vi "TL_init_sCMOS_for_scan.vi"(7 "queue sCMOS":refnum<queue>, 8 "error in":errorcluster, 9 "data":cluster{"Channel":string, "ROI #":i32}, 10 "Channel #":i32, 11 "Time lapse parameters":T2) -> (0 "error out":errorcluster)   [LabVIEW 2015]
uses:
  CONTROLS/Q_camera_element.ctl
  CONTROLS/Q_main_element.ctl
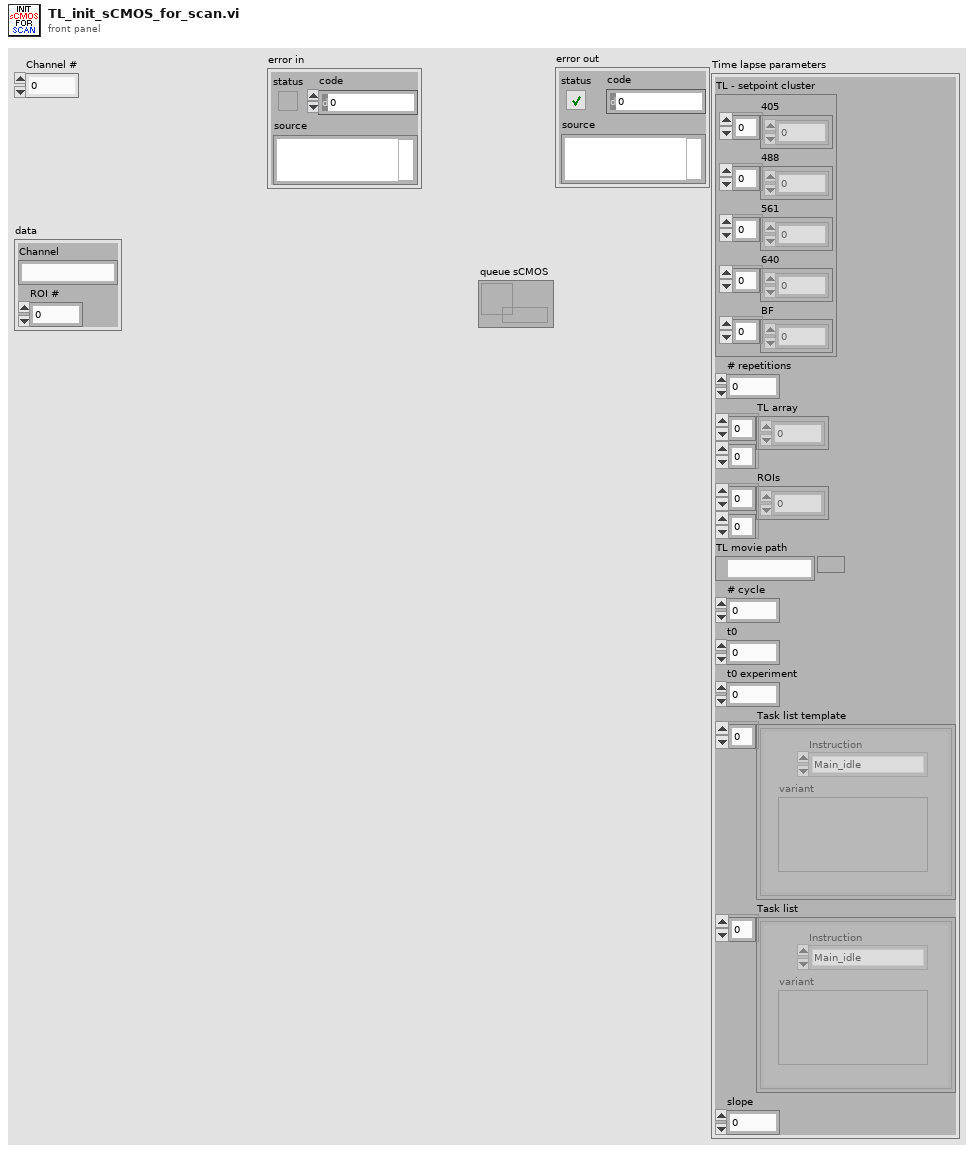
[diagram p1: front panel]
types:
  T1 = typedef "Q_main_element.ctl" = cluster{"variant":variant, "Instruction":enum16{"Main_idle", "Main_initialize", "Main_error", "Main_DAQ_initialization_results", "Main_ASI_initialization_results", "Main_Piezo_initialization_results", "Main_Valve_initialization_results", "Main_Pump_initialization_results", "Main_CAMERA_initialization_results", "Main_DAQ_error", "Main_ASI_error", "Main_Piezo_error", "Main_CAMERA_error", "Main_Valve_error", "Main_Pump_error", "Main_start_acquiring", "Main_not_acquiring", "Main_acquiring", "Main_stop_acquiring", "Main_change_exposure", "Main_define_ROI", "Main_read_kinetic_time", "Main_cooler", "Main_read_temperature", "Main_save_XY", "Main_load_XY", "Main_discard_XY", "Main_move_to_XY", "Main_measure_QPD", "Main_autofocus_calibration", "Main_save_PID", "Main_change_H_valve_position", "Main_two_way_valve", "Main_save_movie", "Main_init_single_scan", "Main_single_scan", "Main_stop_single_scan", "Main_merFISH_illumination_parameters", "Main_merFISH_buffer_probe_list", "Main_merFISH_injections_procedure", "Main_merFISH_save_setpoint", "Main_merFISH_init", "Main_merFISH_start_autofocus", "Main_merFISH_open_close_valve", "Main_merFISH_hybridization", "Main_merFISH_move_to_ROI", "Main_merFISH_wait_stabilization", "Main_merFISH_scan", "Main_merFISH_photobleaching", "Main_merFISH_save", "Main_merFISH_send_email", "Main_merFISH_close", "Main_TL_define_parameters", "Main_TL_init", "Main_TL_start_autofocus", "Main_TL_move_to_ROI", "Main_TL_wait_for_stabilization", "Main_TL_scan", "Main_TL_wait_cycle_end", "Main_TL_close", "Main_STOP"}}
  T2 = cluster{"TL - setpoint cluster":cluster{"405":dbl[], "488":dbl[], "561":dbl[], "640":dbl[], "BF":dbl[]}, "# repetitions":i32, "TL array":dbl[][], "ROIs":dbl[][], "TL movie path":path, "# cycle":i32, "t0":dbl, "t0 experiment":dbl, "Task list template":T1[], "Task list":T1[], "slope":dbl}
  T3 = typedef "Q_ANDOR_element.ctl" = cluster{"variant":variant, "Instruction":enum16{"sCMOS_idle", "sCMOS_initialize", "sCMOS_error", "sCMOS_security_stop", "sCMOS_not_acquiring", "sCMOS_acquiring", "sCMOS_start_acquiring", "sCMOS_stop_acquiring", "sCMOS_change_exposure", "sCMOS_define_ROI", "sCMOS_cooler", "sCMOS_acquire_movie", "sCMOS_init_scan", "sCMOS_check_new_scan_image", "sCMOS_close_scan", "sCMOS_init_merFISH", "sCMOS_start_acquiring_merFISH", "sCMOS_close_scan_merFISH", "sCMOS_close_merFISH", "sCMOS_init_TL", "sCMOS_start_acquiring_TL", "sCMOS_stop_acquiring_TL", "sCMOS_close_TL", "sCMOS_STOP"}}
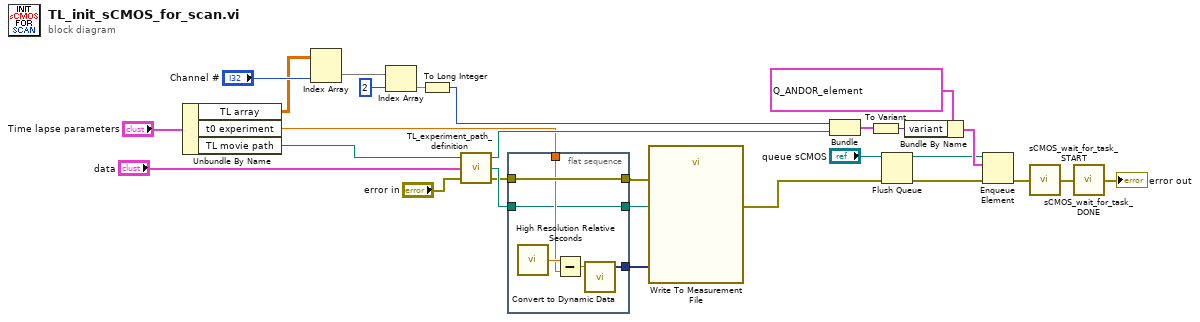
[diagram p0: block diagram]
diagram:
  n1 = Unbundle By Name("Time lapse parameters") -> ("TL array"=w5:dbl[][], "t0 experiment"=w9:dbl, "TL movie path"=w2:path)
  n2 = Index Array(array=w5, index (col)="Channel #") -> (element=w8:dbl[])  [unwired: 1 in]
  n3 = Index Array(array=w8, index=2) -> (element=w4:dbl)
  n4 = To Long Integer(number=w4) -> (32bit integer=w3:i32)
  n5 = call "TL_experiment_path_definition.vi"("error in"="error in", "Path to the time lapse saving folder"="data", "data"=w2) -> ("error out"=w23:errorcluster, "time file path"=w27:path, "movie path"=w21:path)
  n6 = flat-sequence {
    tunnel: w23 -> [w33]
    tunnel: w9 -> [w32]
    tunnel: [w33] -> w25
    tunnel: [w30] -> w24
    tunnel: [w29] -> w26
    tunnel: w27 -> [w29]
    frame #0 {
      n7 = call <vilib>:"High Resolution Relative Seconds.vi"() -> ("relative seconds"=w34:dbl)
      n8 = Subtract(x=w34, y=w32) -> (x-y=w31:dbl)
      n9 = call "Convert to Dynamic Data"("Double"=w31) -> ("Dynamic Data Type"=w30:dynamicdata)  [unwired: 3 in]
    }
  }
  n10 = call "Write To Measurement File"("Signals"=w24, "error in (no error)"=w25, "Filename"=w26) -> ("error out"=w28:errorcluster)  [unwired: 14 in, 2 out]
  n11 = Bundle(w3, "movie path"=w21) -> (w22:cluster{i32, "movie path":path})  [unwired: 1 in]
  n12 = To Variant(anything=w22) -> (Variant=w18:variant)
  n13 = Flush Queue(queue="queue sCMOS", error in (no error)=w28) -> (queue out=w15:refnum<queue>, error out=w14:errorcluster)  [unwired: 1 out]
  n14 = Bundle By Name(cluster=T3 {"variant"=variant, "Instruction"=enum."sCMOS_start_acquiring_TL"} ("Q_ANDOR_element"), "variant"=w18) -> (w19:T3)
  n15 = Enqueue Element(queue=w15, element=w19, error in (no error)=w14) -> (error out=w16:errorcluster)  [unwired: 1 in, 2 out]
  n16 = call "sCMOS_wait_for_task_START.vi"("error in"=w16) -> ("error out"=w17:errorcluster)
  n17 = call "sCMOS_wait_for_task_DONE.vi"("error in"=w17) -> ("error out"=→"error out":errorcluster)
